vi "ReadOutput.vi"(8 "error in (no error)":errorcluster, 11 "TranslationStageActor in":refnum<class "ArduinoTranslationStage.lvclass">) -> (0 "error out":errorcluster, 1 "Output":string, 3 "TranslationStageActor out":refnum<class "ArduinoTranslationStage.lvclass">)   [LabVIEW 2023, in "ArduinoTranslationStage.lvlib" / "ArduinoTranslationStage.lvclass"]
uses:
  ArduinoTranslationStage.lvclass
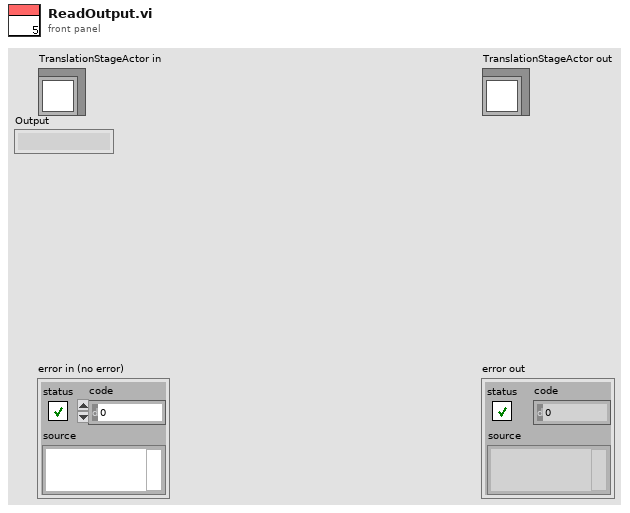
[diagram p1: front panel]
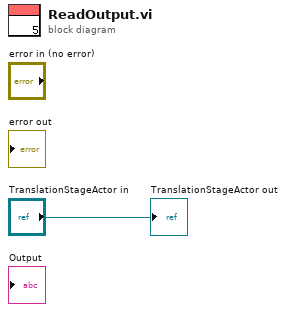
[diagram p0: block diagram]
diagram:
  "TranslationStageActor out" <- "TranslationStageActor in"
